vi "Handle Error.vi"(8 "error in (no error)":errorcluster, 11 "SkynetCompiler in":refnum<class "LVAutomationListener.lvclass">) -> (0 "error out":errorcluster, 2 "stop actor?":bool=TRUE, 3 "SkynetCompiler out":refnum<class "LVAutomationListener.lvclass">)   [LabVIEW 2013, in "LVAutomationListener.lvlib" / "LVAutomationListener.lvclass"]
doc: "(<B>Filename</B>: Actor Framework.lvlib:Actor.lvclass:Handle Error.vi)\n\nDefines how the actor handles an error that occurred while processing a message.\n\nBy default, this method does nothing except stop the actor. This method also treats error code 43 (coming from <B>error in</B>) as a sign that the actor shut down normally. In this situation, the Handle Error method does not return the error on <B>error out</B>, meaning the actor's caller will not receive it. All other error codes will be returned on <B>error out</B>.\n\nA descendant class may override this method to change this behavior."
uses:
  LVAutomationListener.lvclass
  <vilib>/ActorFramework/Actor/Actor.lvclass/Actor.ctl
  <vilib>/ActorFramework/Message Enqueuer/Message Enqueuer.lvclass/Message Enqueuer.ctl
  msgs/Log Event Msg/Log Event Msg.lvclass/Log Event Msg.ctl
  <vilib>/ActorFramework/Message Enqueuer/Init from Existing Queue.vi
  <vilib>/ActorFramework/Message Enqueuer/Enqueue.vi
  <vilib>/ActorFramework/Message Priority Queue/Priority Enqueue.vi
  <vilib>/ActorFramework/Message Enqueuer/Message Enqueuer.lvclass
  msgs/Log Event Msg/Log Event Msg.lvclass
  <vilib>/ActorFramework/Actor/Actor.lvclass
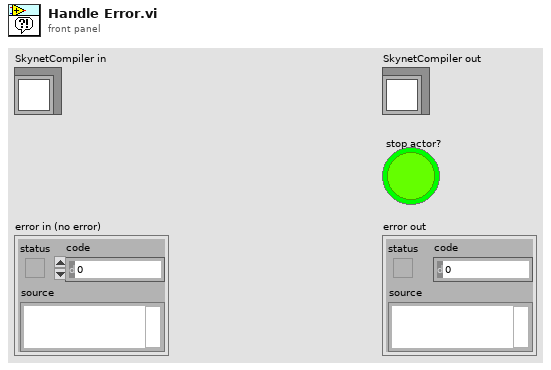
[diagram p1: front panel]
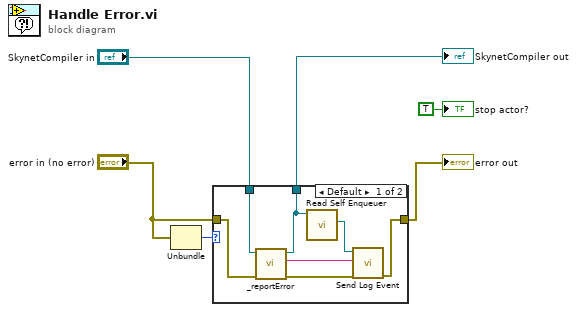
[diagram p0: block diagram]
diagram:
  n1 = Unbundle("error in (no error)") -> ("code"=w5:i32)  [unwired: 2 out]
  n2 = case shown="Default" w5 {
    tunnel: [w9 _] -> w3
    tunnel: "error in (no error)" -> [w10 _]
    tunnel: "SkynetCompiler in" -> [w8 w14]
    tunnel: [w7 w14] -> w1
    frame Default {
      n3 = call "_reportError.vi"("error in (no error)"=w10, "SkynetCompiler in"=w8) -> ("error out"=w11:errorcluster, "Error Text"=w13:string, "SkynetCompiler out"=w7:refnum<class "LVAutomationListener.lvclass">)  [unwired: 7 in]
      n4 = call <vilib>:"Read Self Enqueuer.vi"("Actor"=w7) -> ("Self Enqueuer"=w12:refnum<class "Message Enqueuer.lvclass">)  [unwired: 10 in]
      n5 = call "Send Log Event.vi"("error in (no error)"=w11, "Event Text"=w13, "Message Enqueuer"=w12) -> ("error out"=w9:errorcluster)  [unwired: 7 in, 1 out]
    }
    frame 43 {
      # "\"Cancel Error\" means stop, but \"No Error\" to caller."
    }
  }
  "SkynetCompiler out" <- w1
  "error out" <- w3
  "stop actor?" <- TRUE ("stop actor?")
